vi "Shut_Down_Aero_Tunnel.vi"(3 "Mode":T5=enum."Run VI", 5 "Traverse line In":T2 {"Carrier_2 Q (l/min)" format="%#.2f"; "Row Duration (mins)" format="%#.1f"; "Row No" min=0; "Trace Gas Concentration (%)" min=0.0 format="%#_4f"; "Carrier_1 Q (l/min)" format="%#.4f"; "Start X" format="%#.2f"; "Start Y" format="%#.2f"; "Start Z" format="%#.2f"; "End X" format="%#.2f"; "End Y" format="%#.2f"; "End Z" format="%#.2f"; "Tunnel Speed" format="%#.2f"; "Averaging time (mins)" min=0.0 format="%#.2f"}) -> (0 "Error Message":string, 1 "Status":T1, 2 "Traverse line Out":T2 {"Carrier_2 Q (l/min)" format="%#.2f"; "Row Duration (mins)" format="%#.1f"; "Row No" min=0; "Trace Gas Concentration (%)" min=0.0 format="%#_4f"; "Carrier_1 Q (l/min)" format="%#.4f"; "Start X" format="%#.2f"; "Start Y" format="%#.2f"; "Start Z" format="%#.2f"; "End X" format="%#.2f"; "End Y" format="%#.2f"; "End Z" format="%#.2f"; "Tunnel Speed" format="%#.2f"; "Averaging time (mins)" min=0.0 format="%#.2f"})   [LabVIEW 2021]
uses:
  Gen Trav/Multi_Run_Status.ctl
  ADAM Client/Sub VIs/ADAM Controls/Tunnel_speed_mode.ctl
  ADAM Client/Sub VIs/ADAM Controls/Client_Source_Status.ctl
  Controls/User_Specific_mode.ctl
  Globals/Trav_pos_global.vi
  ADAM Client/Sub VIs/ADAM Controls/Channel_names.ctl
  Globals/Preference_global.vi
  Controls/GMU Gas Line Name.ctl
  Gen Trav/Spacing.ctl
  Gen Trav/Traverse_cluster.ctl
  Controls/Multi_run_mode.ctl
panel:
  # "X           Y          Z"
  # "Start"
  # "End"
  # "X           Y          Z"
  # "Start"
  # "End"
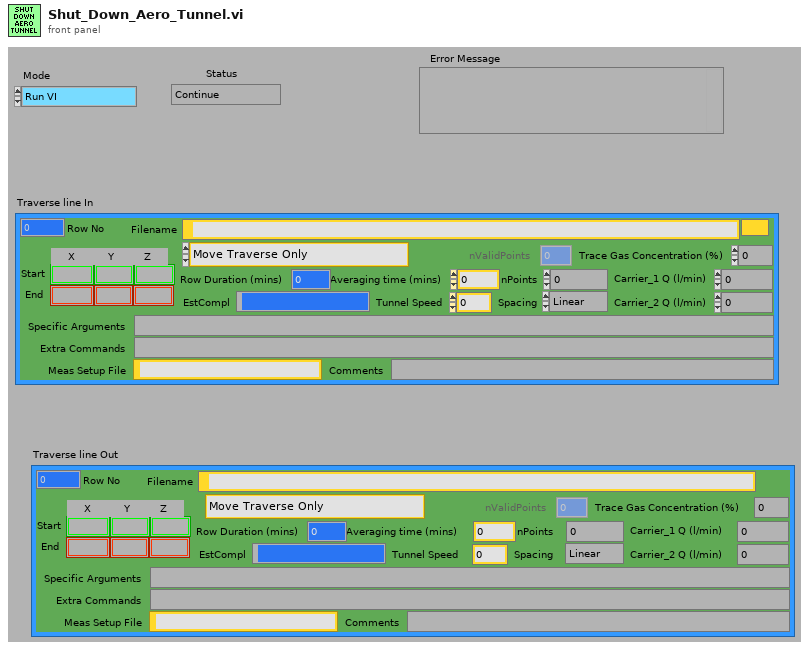
[diagram p1: front panel]
types:
  T1 = typedef "Multi_Run_Status.ctl" = enum16{"Continue", "Continue with Error", "Jump to Next Point", "Jump to Next Row", "Jump To Fall Back", "Terminate Run"}
  T2 = typedef "Traverse_cluster.ctl" = cluster{"Start X":sgl, "Start Y":sgl, "Start Z":sgl, "End X":sgl, "End Y":sgl, "End Z":sgl, "nPoints":i32, "Spacing":T3, "Filename":path, "Tunnel Speed":dbl, "Averaging time (mins)":dbl, "Extra Commands":string, "Carrier_1 Q (l/min)":dbl, "Carrier_2 Q (l/min)":dbl, "Trace Gas Concentration (%)":dbl, "Specific Arguments":string, "Comments":string, "Row No":i32, "Row Type Selector":T4, "EstCompl":string, "Row Duration (mins)":dbl, "nValidPoints":i32, "Meas Setup File":string}
  T3 = typedef "Spacing.ctl" = enum16{"Linear", "Log", "Gauss", "Specified", "N/A"}
  T4 = typedef "Multi_run_mode.ctl" = enum16{"Move Traverse Only", "Set Tunnel Speed Only", "Set Source Only", "Set Measurement Conditions", "Single Measurement", "Vertical Profile", "Lateral Profile", "Longitudinal Profile", "Multi-Axis Profile", "Explore Volume", "Auto Calibrate", "Meas Fast FID Bkgnd", "Check Beam Power", "Scanning Valve Measurement", "Run VI Named:", "Set ADAM Ch", "Wait (minutes)", "Send Message", "Synchronize With:", "Fall Back to this Row", "Turn Off Row Repeating", "Traverse 3D Volume", "Blank Row", "Jump to Fall Back Row"}
  T5 = typedef "User_Specific_mode.ctl" = enum16{"Check VI only", "Run VI"}
  T6 = typedef "GMU Gas Line Name.ctl" = enum16{"GMU1 Source", "GMU2 Source", "GMU2 Calib", "CPP GRC-A", "CPP GRC-B"}
  T7 = typedef "Channel_names.ctl" = enum16{"Active Only", "Active + Off", "All Channels", "Changeable Only"}
  T8 = typedef "Client_Source_Status.ctl" = enum16{"Not Using", "Using", "Must Have"}
  T9 = typedef "Tunnel_speed_mode.ctl" = enum16{"Set Speed", "Set Speed then wait", "Is tunnel speed allowable?"}
  T10 = cluster{"second":i32, "minute":i32, "hour":i32, "day of month":i32, "month":i32, "year":i32, "day of week":i32, "day of year":i32, "is DST":i32}
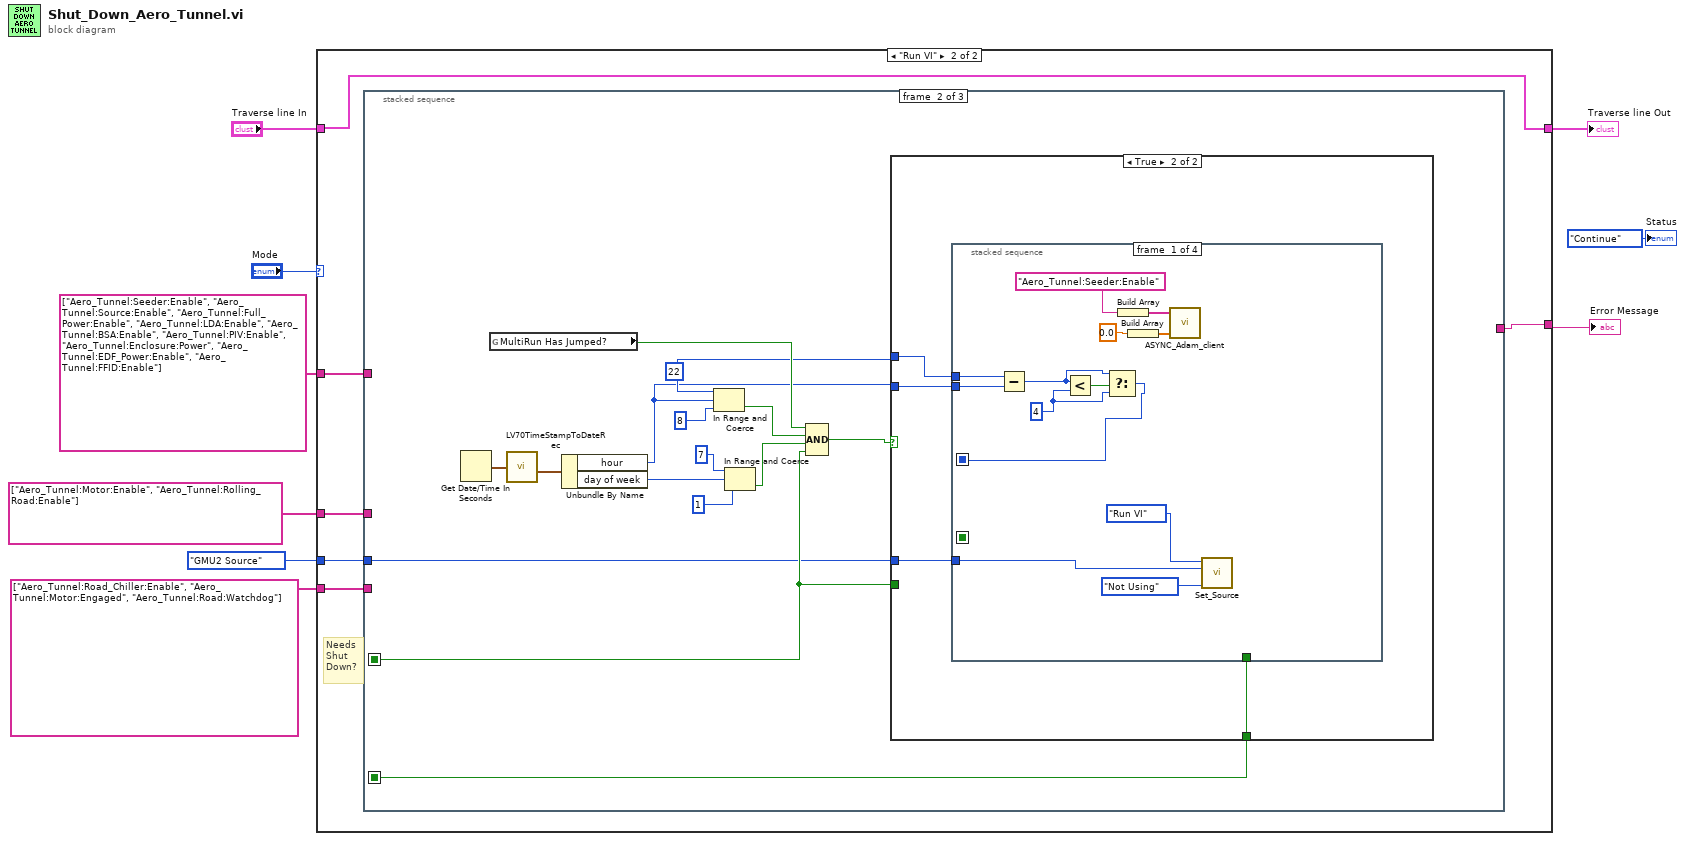
[diagram p0: block diagram]
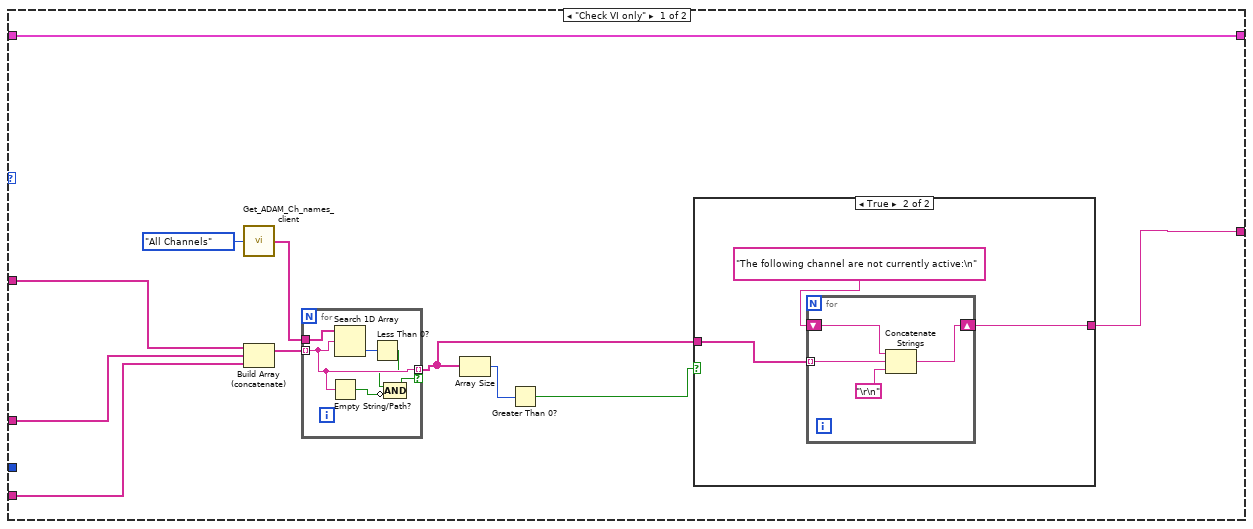
[diagram p2: hidden frame]
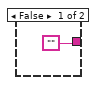
[diagram p3: hidden frame]
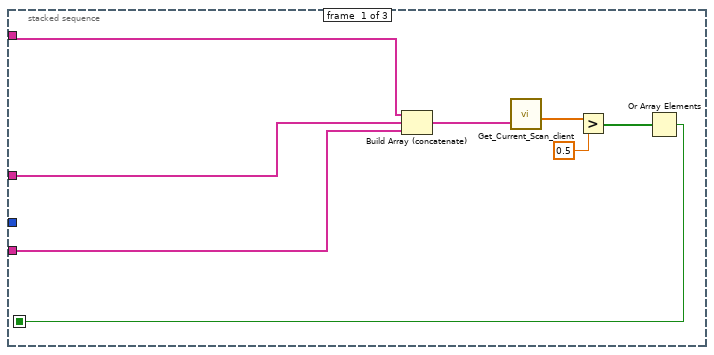
[diagram p4: hidden frame]
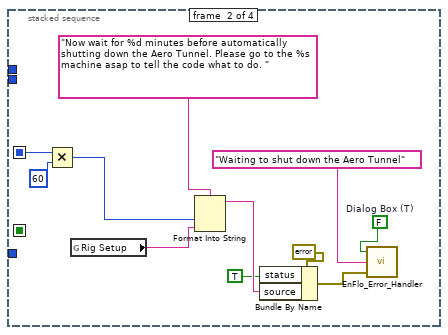
[diagram p6: hidden frame]
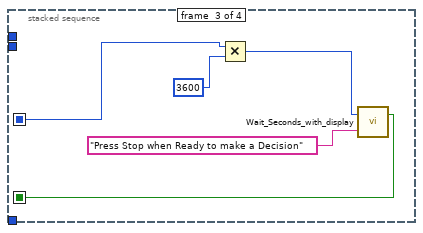
[diagram p7: hidden frame]
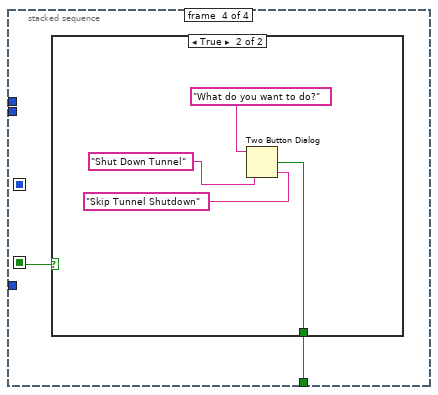
[diagram p8: hidden frame]
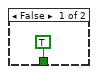
[diagram p9: hidden frame]
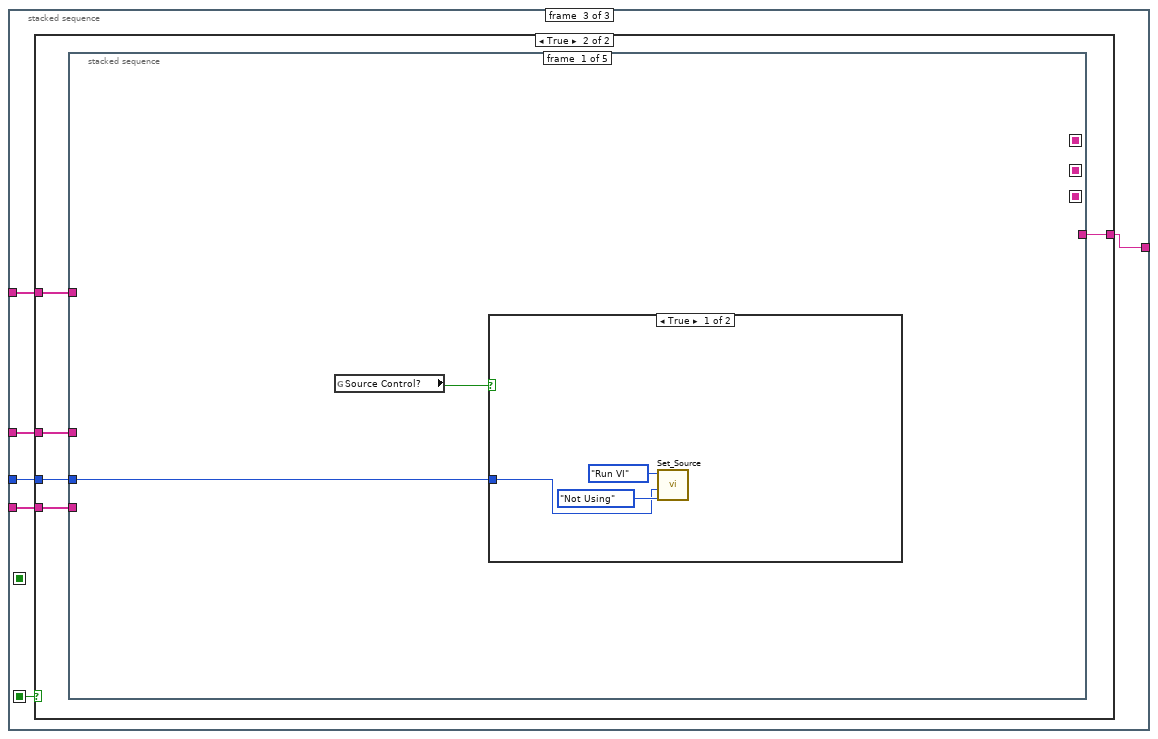
[diagram p10: hidden frame]
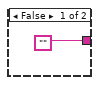
[diagram p11: hidden frame]
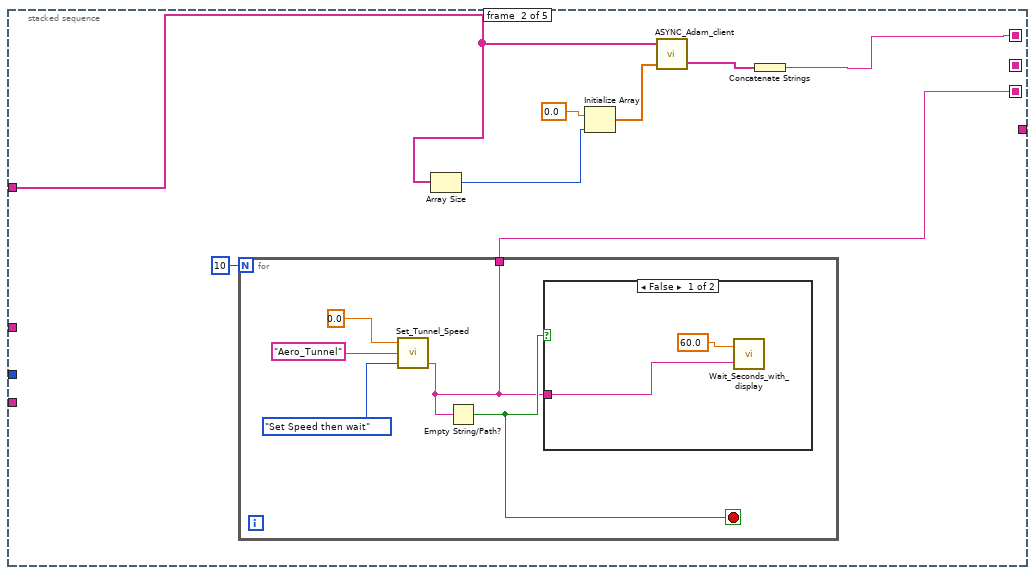
[diagram p13: hidden frame]
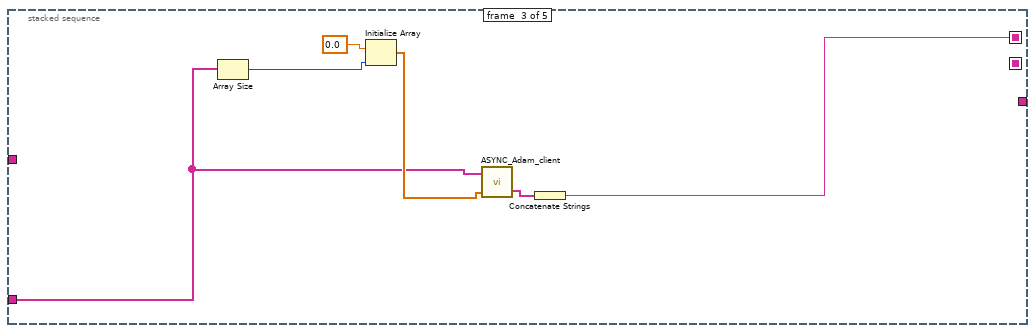
[diagram p15: hidden frame]
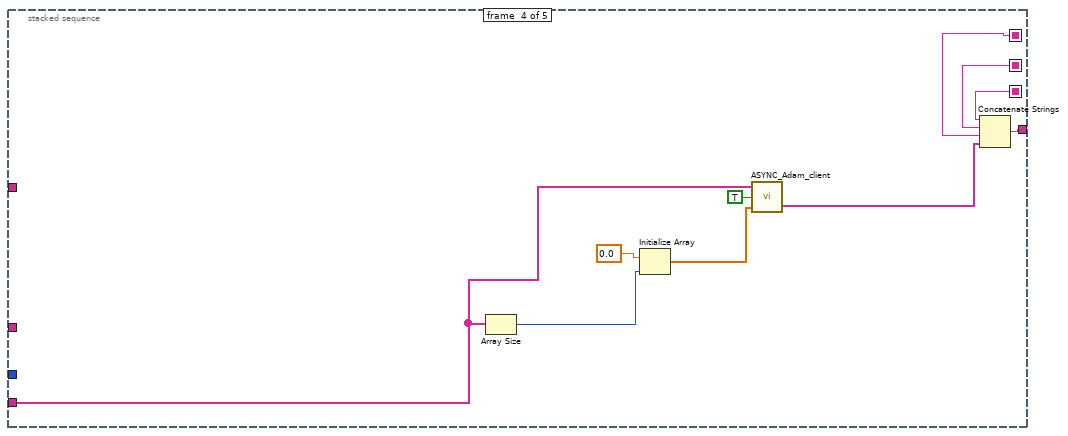
[diagram p16: hidden frame]
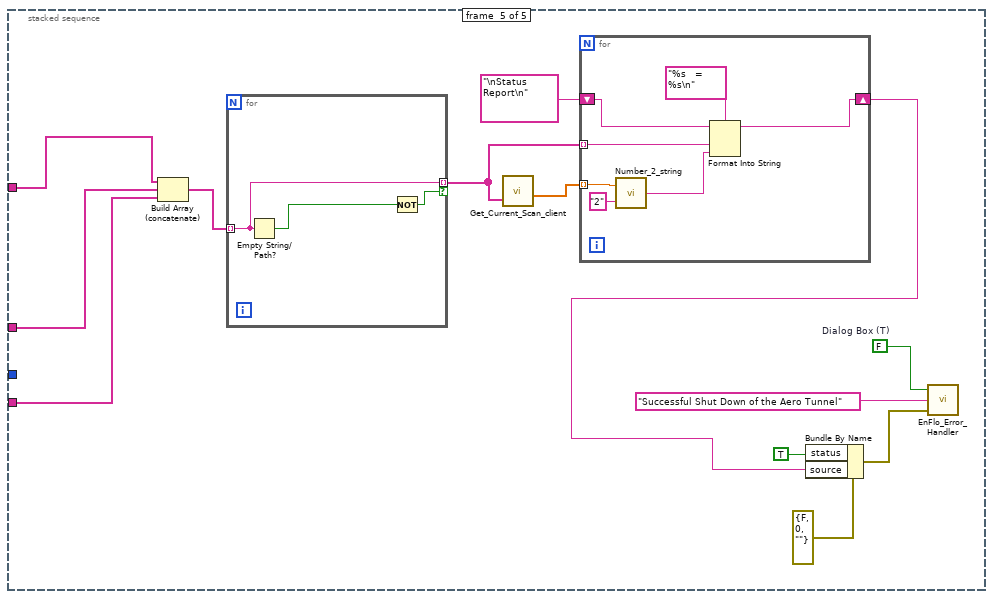
[diagram p17: hidden frame]
diagram:
  n1 = case shown="\"Run VI\"" "Mode" {
    tunnel: "Traverse line In" -> [w20 w40]
    tunnel: [w20 w40] -> w7
    tunnel: [w14 w36] -> w6
    tunnel: string[] ["Aero_Tunnel:Seeder:Enable", "Aero_Tunnel:Source:Enable", "Aero_Tunnel:Full_Power:Enable", "Aero_Tunnel:LDA:Enable", "Aero_Tunnel:BSA:Enable", "Aero_Tunnel:PIV:Enable", "Aero_Tunnel:Enclosure:Power", "Aero_Tunnel:EDF_Power:Enable", "Aero_Tunnel:FFID:Enable"] ("appended array") -> [w19 w39]
    tunnel: string[] ["Aero_Tunnel:Road_Chiller:Enable", "Aero_Tunnel:Motor:Engaged", "Aero_Tunnel:Road:Watchdog"] ("appended array") -> [w17 w38]
    tunnel: string[] ["Aero_Tunnel:Motor:Enable", "Aero_Tunnel:Rolling_Road:Enable"] ("appended array") -> [w18 w37]
    tunnel: GMU_Gas_Line_Name."GMU2 Source" ("Gas Line Name") -> [_ w35]
    frame "Check VI only" {
      n2 = call "Get_ADAM_Ch_names_client.vi"("Channel names set"=Channel_names."All Channels") -> ("Ch names"=w13:string[])
      n3 = Build Array (concatenate)(w19, w18, w17) -> (w12:string[])
      n4 = for {
        tunnel: w13 -> [w34]
        tunnel: w12 -> [w32] mode=indexing
        tunnel: [w32] -> w15 mode=indexing if=w29
        n5 = Empty String/Path?(string/path=w32) -> (empty?=w30:bool)
        n6 = Search 1D Array(1D array=w34, element=w32) -> (index of element=w33:i32)  [unwired: 1 in]
        n7 = Less Than 0?(x=w33) -> (x < 0?=w31:bool)
        n8 = Compound Arithmetic op=AND(w31, invert w30) -> (w29:bool)
      }
      n9 = Array Size(array=w15) -> (size(s)=w10:i32)
      n10 = Greater Than 0?(x=w10) -> (x > 0?=w11:bool)
      n11 = case shown="True" w11 {
        tunnel: w15 -> [_ w24]
        tunnel: ["" w22] -> w14
        frame False {
        }
        frame True {
          n12 = for {
            tunnel: w24 -> [w27] mode=indexing
            shift-right: [w25] -> w22
            shift-left: "The following channel are not currently active:\n" -> [w26]
            n13 = Concatenate Strings(w26, w27, "\r\n") -> (w25:string)
          }
        }
      }
    }
    frame "Run VI" {
      # "Needs\nShut\nDown?"
      n14 = stacked-sequence {
        seq-local: [_ w51 _] -> [_ _ w106]
        seq-local: [w41 _ _] -> [_ w50 _]
        tunnel: w39 -> [w44 _ w110]
        tunnel: w38 -> [w42 _ w109]
        tunnel: w37 -> [w43 _ w108]
        tunnel: [_ _ w107] -> w36
        tunnel: w35 -> [_ w49 w105]
        frame #0 {
          n15 = Build Array (concatenate)(w44, w43, w42) -> (w45:string[])
          n16 = call "Get_Current_Scan_client.vi"("multipleChannels"=w45) -> ("Numerical Values"=w46:dbl[])  [unwired: 1 in, 3 out]
          n17 = Greater?(x=w46, y=0.5) -> (0:w48:bool[])
          n18 = Or Array Elements(Boolean array=w48) -> (logical OR=w41:bool)
        }
        frame #1 {
          w53 = 22 ("lower limit")
          n19 = Get Date/Time In Seconds() -> (seconds since 1Jan1904=w60:timestamp)
          n20 = global read "Trav_pos_global.vi" "MultiRun Has Jumped?"() -> (w55:bool)
          n21 = call <vilib>:"LV70TimeStampToDateRec.vi"("time stamp"=w60) -> ("date time rec"=w63:T10)
          n22 = Unbundle By Name(w63) -> ("hour"=w52:i32, "day of week"=w59:i32)
          n23 = In Range and Coerce(upper limit=w53, x=w52, lower limit=8) -> (In Range?=w56:bool)  [unwired: 1 out]
          n24 = In Range and Coerce(upper limit=7, x=w59, lower limit=1) -> (In Range?=w57:bool)  [unwired: 1 out]
          n25 = Compound Arithmetic op=AND(w55, w56, w57, w50) -> (w54:bool)
          n26 = case shown="True" w54 {
            tunnel: w53 -> [_ w68]
            tunnel: w52 -> [_ w67]
            tunnel: [w64 w66] -> w51
            tunnel: w50 -> [w64 _]
            tunnel: w49 -> [_ w65]
            frame False {
            }
            frame True {
              n27 = stacked-sequence {
                seq-local: [_ _ w94 _] -> [_ _ _ w98]
                seq-local: [w70 _ _ _] -> [_ w82 w93 _]
                tunnel: w68 -> [w81 _ _ _]
                tunnel: w67 -> [w80 _ _ _]
                tunnel: [_ _ _ w99] -> w66
                tunnel: w65 -> [w69 _ _ _]
                frame #0 {
                  w77 = 4 ("y")
                  n28 = Subtract(x=w81, y=w80) -> (x-y=w78:i32)
                  n29 = Less?(x=w78, y=w77) -> (x < y?=w79:bool)
                  n30 = Select(t=w78, s=w79, f=w77) -> (s? t:f=w70:i32)
                  n31 = Build Array("Aero_Tunnel:Seeder:Enable") -> (w73:string[])
                  n32 = Build Array(0.0 ("element")) -> (w72:dbl[])
                  n33 = call "ASYNC_Adam_client.vi"("Values"=w72, "Channel Names"=w73) -> ()  [unwired: 1 in, 2 out]
                  n34 = call "Set_Source.vi"("Source Status"=Client_Source_Status."Not Using", "Gas Line Name"=w69, "Simulate/Run"=User_Specific_mode."Run VI") -> ()  [unwired: 2 in, 6 out]
                }
                frame #1 {
                  w85 = FALSE  # Dialog Box (T)
                  n35 = Multiply(x=w82, y=60) -> (x*y=w90:i32)
                  n36 = global read "Preference_global.vi" "Rig Setup"() -> (w91:string)
                  n37 = Format Into String(format string="Now wait for %d minutes before automatically shutting down the Aero Tunnel. Please go to the %s machine asap to tell the code what to do. ", w90, w91) -> (resulting string=w92:string)  [unwired: 2 in, 1 out]
                  n38 = Bundle By Name(cluster=errorcluster {"status"=FALSE, "code"=0, "source"=""} ("error in (no error)"), "status"=TRUE ("Bundle Element"), "source"=w92) -> (w83:errorcluster)
                  n39 = call "EnFlo_Error_Handler.vi"("error in (no error)"=w83, "Error Type"="Waiting to shut down the Aero Tunnel", "Dialog Box (F)"=w85) -> ()  [unwired: 3 out]
                }
                frame #2 {
                  n40 = Multiply(x=w93, y=3600) -> (x*y=w95:i32)
                  n41 = call "Wait_Seconds_with_display.vi"("Message"="Press Stop when Ready to make a Decision", "Seconds to wait"=w95) -> ("Stopped"=w94:bool)  [unwired: 1 out]
                }
                frame #3 {
                  n42 = case shown="True" w98 {
                    tunnel: [TRUE ("T button?") w101] -> w99
                    frame False {
                    }
                    frame True {
                      n43 = Two Button Dialog(message="What do you want to do?", 1:"Skip Tunnel Shutdown" ("F button name (\"Cancel\")"), 2:"Shut Down Tunnel" ("T button name (\"OK\")")) -> (T button?=w101:bool)
                    }
                  }
                }
              }
            }
          }
        }
        frame #2 {
          n44 = case shown="True" w106 {
            tunnel: w110 -> [_ w116]
            tunnel: w109 -> [_ w115]
            tunnel: w108 -> [_ w114]
            tunnel: ["" w113] -> w107
            tunnel: w105 -> [_ w112]
            frame False {
            }
            frame True {
              n45 = stacked-sequence {
                seq-local: [_ w125 _ _ _] -> [_ _ _ w147 _]
                seq-local: [_ _ w137 _ _] -> [_ _ _ w148 _]
                seq-local: [_ w122 _ _ _] -> [_ _ _ w143 _]
                tunnel: w116 -> [_ w124 _ _ w160]
                tunnel: w115 -> [_ _ _ w149 w162]
                tunnel: w114 -> [_ _ w139 _ w161]
                tunnel: [_ _ _ w145 _] -> w113
                tunnel: w112 -> [w117 _ _ _ _]
                frame #0 {
                  n46 = global read "Trav_pos_global.vi" "Source Control?"() -> (w118:bool)
                  n47 = case shown="True" w118 {
                    tunnel: w117 -> [w119 _]
                    frame True {
                      n48 = call "Set_Source.vi"("Source Status"=Client_Source_Status."Not Using", "Gas Line Name"=w119, "Simulate/Run"=User_Specific_mode."Run VI") -> ()  [unwired: 2 in, 6 out]
                    }
                    frame False {
                    }
                  }
                }
                frame #1 {
                  n49 = for {
                    N: 10 -> [_]
                    tunnel: [w131] -> w122
                    stop <- w132 stop-if-true
                    n50 = call "Set_Tunnel_Speed.vi"("Mode"=Tunnel_speed_mode."Set Speed then wait", "Rig Name (default Empty)"="Aero_Tunnel", "Tunnel Velocity m/s"=0.0) -> ("Error String"=w131:string)  [unwired: 1 in, 1 out]
                    n51 = Empty String/Path?(string/path=w131) -> (empty?=w132:bool)
                    n52 = case shown="False" w132 {
                      tunnel: w131 -> [w135 _]
                      frame False {
                        n53 = call "Wait_Seconds_with_display.vi"("Message"=w135, "Seconds to wait"=60.0) -> ()  [unwired: 2 out]
                      }
                      frame True {
                      }
                    }
                  }
                  n54 = Array Size(array=w124) -> (size(s)=w129:i32)
                  n55 = Initialize Array(0.0 ("Input Element"), w129) -> (w128:dbl[])
                  n56 = call "ASYNC_Adam_client.vi"("Values"=w128, "Channel Names"=w124) -> ("Scan Comments"=w126:string[])  [unwired: 1 in, 1 out]
                  n57 = Concatenate Strings(w126) -> (w125:string)
                }
                frame #2 {
                  n58 = Array Size(array=w139) -> (size(s)=w142:i32)
                  n59 = Initialize Array(0.0 ("Input Element"), w142) -> (w140:dbl[])
                  n60 = call "ASYNC_Adam_client.vi"("Values"=w140, "Channel Names"=w139) -> ("Scan Comments"=w138:string[])  [unwired: 1 in, 1 out]
                  n61 = Concatenate Strings(w138) -> (w137:string)
                }
                frame #3 {
                  n62 = Array Size(array=w149) -> (size(s)=w152:i32)
                  n63 = Initialize Array(0.0 ("Input Element"), w152) -> (w151:dbl[])
                  n64 = call "ASYNC_Adam_client.vi"("Values"=w151, "Check Value is in the scan table?"=TRUE, "Channel Names"=w149) -> ("Scan Comments"=w146:string[])  [unwired: 1 out]
                  n65 = Concatenate Strings(w143, w148, w147, w146) -> (w145:string)
                }
                frame #4 {
                  w157 = FALSE  # Dialog Box (T)
                  n66 = Build Array (concatenate)(w160, w161, w162) -> (w159:string[])
                  n67 = for {
                    tunnel: w159 -> [w166] mode=indexing
                    tunnel: [w166] -> w158 mode=indexing if=w167
                    n68 = Empty String/Path?(string/path=w166) -> (empty?=w168:bool)
                    n69 = Not(x=w168) -> (.not. x?=w167:bool)
                  }
                  n70 = call "Get_Current_Scan_client.vi"("multipleChannels"=w158) -> ("Numerical Values"=w163:dbl[])  [unwired: 1 in, 3 out]
                  n71 = for {
                    tunnel: w158 -> [w175] mode=indexing
                    shift-right: [w172] -> w164
                    shift-left: "\nStatus Report\n" -> [w173]
                    tunnel: w163 -> [w171] mode=indexing
                    n72 = call "Number_2_string.vi"("precision"="2", "number"=w171) -> ("String"=w169:string)
                    n73 = Format Into String(format string="%s   =  %s\n", initial string=w173, w175, w169) -> (resulting string=w172:string)  [unwired: 1 in, 1 out]
                  }
                  n74 = Bundle By Name(cluster=errorcluster {"status"=FALSE, "code"=0, "source"=""} ("error in (no error)"), "status"=TRUE ("Bundle Element"), "source"=w164) -> (w156:errorcluster)
                  n75 = call "EnFlo_Error_Handler.vi"("error in (no error)"=w156, "Error Type"="Successful Shut Down of the Aero Tunnel", "Dialog Box (F)"=w157) -> ()  [unwired: 3 out]
                }
              }
            }
          }
        }
      }
    }
  }
  "Traverse line Out" <- w7
  "Error Message" <- w6
  "Status" <- Multi_Run_Status."Continue" ("Status")
